vi "ClimbExecute.vi"(8 "error in (no error)":errorcluster) -> (0 "error out":errorcluster)   [LabVIEW 2023]
uses:
  <vilib>/Rock Robotics/WPI/ThirdParty/REV Robotics/REVLib/SubVI/Public/SPARK Get Encoder Status Position.vi
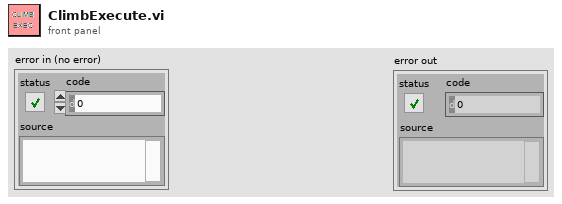
[diagram p1: front panel]
types:
  T1 = typedef "WPI_SwitchDevRef.ctl" = cluster{"DevStatus":errorcluster, "DIO Channel":T2, "CntIndex":T3, "Normally Closed":bool}
  T2 = typedef "FPGA_DIOChannel.ctl" = enum8{"DIO 0", "DIO 1", "DIO 2", "DIO 3", "DIO 4", "DIO 5", "DIO 6", "DIO 7", "DIO 8", "DIO 9", "DIO MXP 0", "DIO MXP 1", "DIO MXP 2", "DIO MXP 3", "DIO MXP 4", "DIO MXP 5", "DIO MXP 6", "DIO MXP 7", "DIO MXP 8", "DIO MXP 9", "DIO MXP 10", "DIO MXP 11", "DIO MXP 12", "DIO MXP 13", "DIO MXP 14", "DIO MXP 15", "SPI Port CS1", "SPI Port CS2", "SPI Port CS3", "SPI Port MISO", "SPI Port MOSI", "Invalid"}
  T3 = typedef "FPGA_CounterCtrSystemIndex.ctl" = enum8{"Ctr 0", "Ctr 1", "Ctr 2", "Ctr 3", "Ctr 4", "Ctr 5", "Ctr 6", "Ctr 7", "Invalid"}
  T4 = typedef "WPI_MotorControlDeviceRef.ctl" = cluster{"DeviceStatus":errorcluster, "Type":T5, "PWM":cluster{"PWM Channel":T6, "DeadBand":T7}, "CAN":cluster{"Device Number":u8, "SetOutput VI Ref":variant, "GetOutput VI Ref":variant, "Enable VI Ref":variant, "Disable VI Ref":variant, "Data":variant}, "Invert":bool, "DIO PWM":cluster{"PWM \"Enable\" Channel":T6, "DIOChannel":T2, "PWM Rate":dbl}}
  T5 = typedef "WPI_MotorControlType.ctl" = enum16{"PWM", "CAN", "DIO PWM"}
  T6 = typedef "FPGA_DIOPWMChannel.ctl" = enum8{"PWM 0", "PWM 1", "PWM 2", "PWM 3", "PWM 4", "PWM 5", "PWM 6", "PWM 7", "PWM 8", "PWM 9", "PWM MXP 0", "PWM MXP 1", "PWM MXP 2", "PWM MXP 3", "PWM MXP 4", "PWM MXP 5", "PWM MXP 6", "PWM MXP 7", "PWM MXP 8", "PWM MXP 9", "Invalid"}
  T7 = typedef "WPI_PWMDeadband.ctl" = cluster{"Name":string, "maxPositivePwm":i32, "minPositivePwm":i32, "centerPwm":i32, "maxNegativePwm":i32, "minNegativePwm":i32, "angularRange":u16}
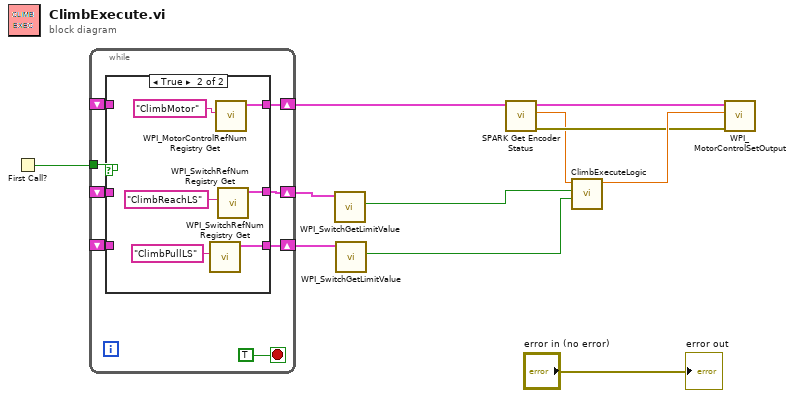
[diagram p0: block diagram]
diagram:
  n1 = First Call?() -> (First Call?: T/F=w11:bool)
  n2 = while {
    tunnel: w11 -> [w18]
    shift-right: [w17] -> w4
    shift-left: _ -> [w16]
    shift-right: [w15] -> w8
    shift-left: _ -> [w13]
    shift-right: [w14] -> w7
    shift-left: _ -> [w12]
    stop <- TRUE stop-if-true
    n3 = case shown="True" w18 {
      tunnel: [w22 w27] -> w17
      tunnel: w16 -> [w22 _]
      tunnel: [w21 w24] -> w15
      tunnel: [w20 w23] -> w14
      tunnel: w13 -> [w21 _]
      tunnel: w12 -> [w20 _]
      frame False {
      }
      frame True {
        n4 = call <vilib>:"WPI_SwitchRefNum Registry Get.vi"("refnum name"="ClimbPullLS") -> ("SwitchDevRef"=w23:T1)  [unwired: 9 in, 1 out]
        n5 = call <vilib>:"WPI_MotorControlRefNum Registry Get.vi"("refnum name"="ClimbMotor") -> ("MotorControlDevRef"=w27:T4)  [unwired: 9 in, 1 out]
        n6 = call <vilib>:"WPI_SwitchRefNum Registry Get.vi"("refnum name"="ClimbReachLS") -> ("SwitchDevRef"=w24:T1)  [unwired: 9 in, 1 out]
      }
    }
  }
  n7 = call <vilib>:"WPI_SwitchGetLimitValue.vi"("SwitchDevRef"=w8) -> ("Switch Pressed"=w6:bool)  [unwired: 8 in, 2 out]
  n8 = call <vilib>:"WPI_SwitchGetLimitValue.vi"("SwitchDevRef"=w7) -> ("Switch Pressed"=w5:bool)  [unwired: 8 in, 2 out]
  n9 = call-poly <vilib>:"SPARK Get Encoder Status.vi"("MotorControlDevRef in"=w4) -> ("error out"=w2:errorcluster, "Sensor Position"=w1:dbl, "MotorControlDevRef out"=w3:T4)  [unwired: 7 in, 1 out]
  n10 = call "ClimbExecuteLogic.vi"("Rev"=w5, "Fwd"=w6, "SensorPosition"=w1) -> ("MotorDemand"=w10:dbl)  [unwired: 6 in, 2 out]
  n11 = call <vilib>:"WPI_MotorControlSetOutput.vi"("error in (no error)"=w2, "Output"=w10, "MotorControlDevRef"=w3) -> ()  [unwired: 6 in, 3 out]
  "error out" <- "error in (no error)"
